vi "Read Channel Type.vi"(8 "error in":errorcluster, 11 "Plugin_Channels in":refnum<class "Plugin_Channels.lvclass">) -> (0 "error out":errorcluster, 2 "Channel Type":T1, 3 "Plugin_Channels out":refnum<class "Plugin_Channels.lvclass">)   [LabVIEW 2020, in "Plugin.lvlib" / "Plugin_Channels.lvclass"]
doc: "Reads the channel type."
uses:
  Plugin_Channels.lvclass
  Typedefs/Channel Type.ctl
  Plugin_Channels.lvclass/Plugin_Channels.ctl
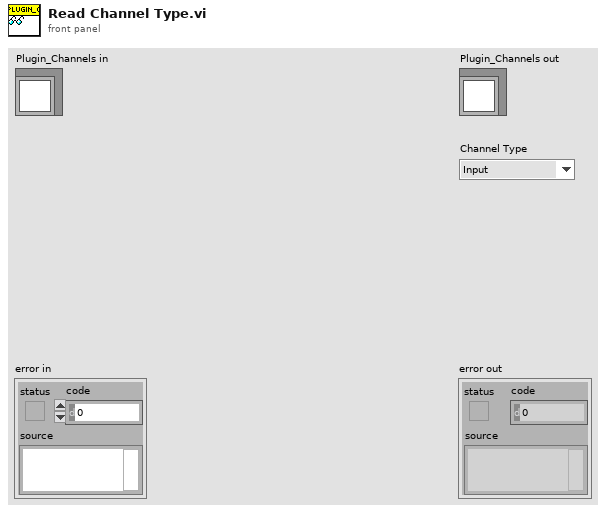
[diagram p1: front panel]
types:
  T1 = typedef "Plugin.lvlib/Plugin_Channels.lvclass/Channel Type.ctl" = enum16{"Input", "Output"}
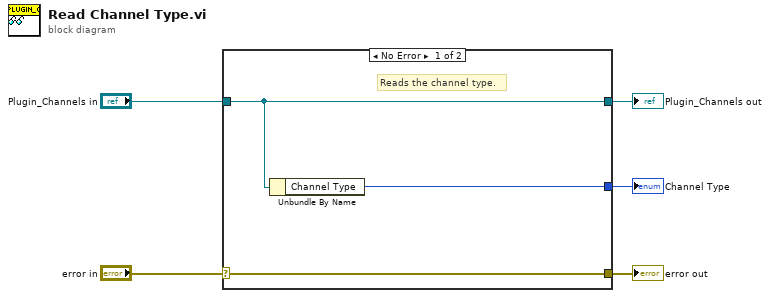
[diagram p0: block diagram]
diagram:
  n1 = case shown="No Error" "error in" {
    selector: "error in" -> [w8 w9]
    tunnel: [w8 w9] -> w4
    tunnel: [w7 w10] -> w2
    tunnel: "Plugin_Channels in" -> [w7 w10]
    tunnel: [w6 _] -> w1
    frame No Error {
      # "Reads the channel type."
      n2 = Unbundle By Name(w7) -> ("Channel Type"=w6:T1)
    }
    frame Error {
    }
  }
  "error out" <- w4
  "Plugin_Channels out" <- w2
  "Channel Type" <- w1
